vi "Read L2 Filter.vi"(8 "error in (no error)":errorcluster, 11 "L2Enet_RW_CORE in":refnum<class "L2ENET_RW_CORE.lvclass">) -> (0 "error out":errorcluster, 2 "L2 Filter":T1[](array[typedef]) {"EtherType" format="%04x"; "SMAC" format="%02x"; "DMAC" format="%02x"}, 3 "L2Enet_RW_CORE out":refnum<class "L2ENET_RW_CORE.lvclass">)   [LabVIEW 2021, in "L2ENET_RW_CORE.lvclass"]
uses:
  L2ENET_RW_CORE.lvclass
  L2ENET_RW_CORE.lvclass/L2ENET_RW_CORE.ctl
  <vilib>/CIF Foundation/CIF Enet Parse and Build/typedef/L2 & L3/L2 Filter.ctl
  <vilib>/CIF Foundation/CIF Enet Parse and Build/Ethernet_Parse_Build_CIF.lvlib
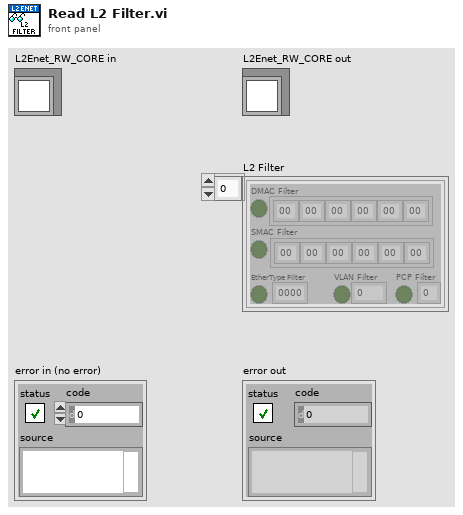
[diagram p1: front panel]
types:
  T1 = typedef "Ethernet_Parse_Build_CIF.lvlib/L2 Filter.ctl" = cluster{"DMAC":u8[], "DMAC Filter":bool, "SMAC":u8[], "SMAC Filter":bool, "EtherType":u16, "EtherType Filter":bool, "VLAN":u16, "VLAN Filter":bool, "PCP":u8, "PCP Filter":bool}
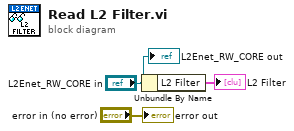
[diagram p0: block diagram]
diagram:
  n1 = Unbundle By Name("L2Enet_RW_CORE in") -> ("L2 Filter"=→"L2 Filter":T1[])
  "error out" <- "error in (no error)"
  "L2Enet_RW_CORE out" <- "L2Enet_RW_CORE in"
